vi "zipMultiFiles.vi"(9 "Source Files":string[](array[string]), 10 "zip folderFile":path, 11 "Source path":path) -> (0 "error out":errorcluster)   [LabVIEW 2012]
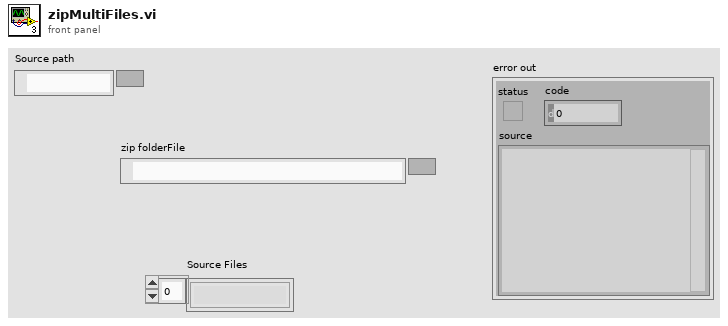
[diagram p1: front panel]
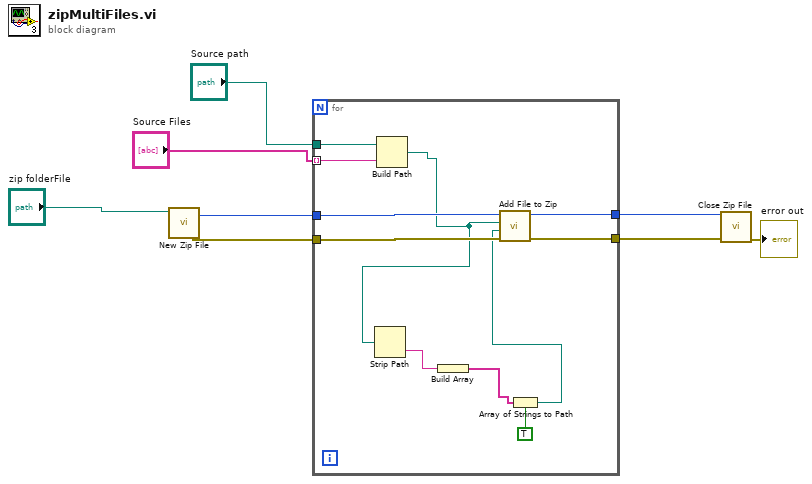
[diagram p0: block diagram]
diagram:
  n1 = call <vilib>:"New Zip File.vi"("target"="zip folderFile") -> ("error out"=w4:errorcluster, "zip file out"=w8:i64)  [unwired: 4 in, 1 out]
  n2 = for {
    tunnel: w8 -> [w19]
    tunnel: [w18] -> w7
    tunnel: [w17] -> w6
    tunnel: w4 -> [w16]
    tunnel: "Source path" -> [w11]
    tunnel: "Source Files" -> [w10] mode=indexing
    n3 = Build Path(base path=w11, name or relative path=w10) -> (appended path=w9:path)
    n4 = Strip Path(path=w9) -> (name=w13:string)  [unwired: 1 out]
    n5 = Build Array(w13) -> (w12:string[])
    n6 = Array of Strings to Path(0:w12, 1:TRUE ("relative")) -> (2:w14:path)
    n7 = call <vilib>:"Add File to Zip.vi"("error in (no error)"=w16, "destination path in zip"=w14, "source file path"=w9, "zip file in"=w19) -> ("error out"=w18:errorcluster, "zip file out"=w17:i64)  [unwired: 6 in]
  }
  n8 = call <vilib>:"Close Zip File.vi"("error in (no error)"=w7, "zip file in"=w6) -> ("error out"=→"error out":errorcluster)  [unwired: 5 in]
